vi "PH_IEEE1394Camera.get Bus Type.vi"(1 "Camera Attributes":T1[](array[typedef])) -> (0 "Bus Type":string)   [LabVIEW 2014, in "PH_IEEE1394Camera.lvlib"]
uses:
  PH_IEEE1394Camera.lvlib
  PH_IEEE1394Camera.Cam Attribute.ctl
  <vilib>/vision/driver/IMAQdx.llb/IMAQdx Attribute Type.ctl
  <vilib>/vision/driver/NI_Vision_Acquisition_Software.lvlib
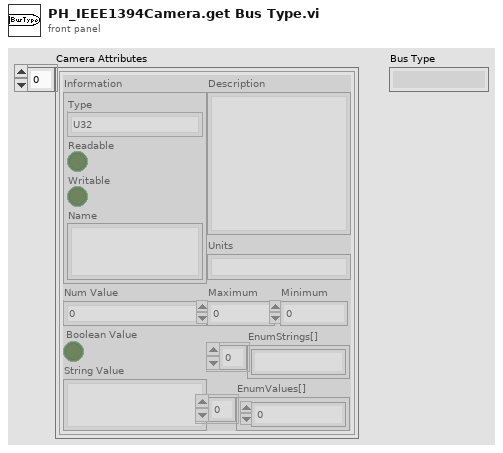
[diagram p1: front panel]
types:
  T1 = typedef "PH_IEEE1394Camera.lvlib/PH_IEEE1394Camera.Cam Attribute.ctl" = cluster{"Information":cluster{"Type":T2, "Readable":bool, "Writable":bool, "Name":string}, "Num Value":dbl, "String Value":string, "Maximum":dbl, "Minimum":dbl, "Units":string, "Description":string, "EnumStrings[]":string[], "EnumValues[]":u32[], "Boolean Value":bool}
  T2 = typedef "NI_Vision_Acquisition_Software.lvlib/IMAQdx Attribute Type.ctl" = enum32{"U32", "I64", "DBL", "String", "Enum", "Bool", "Command"}
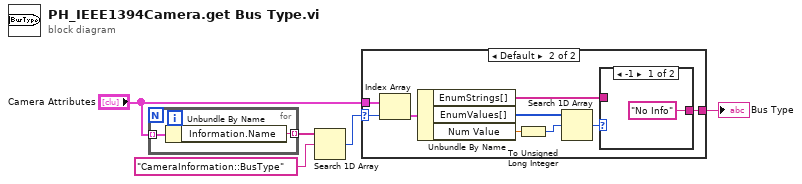
[diagram p0: block diagram]
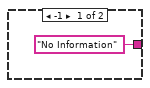
[diagram p2: hidden frame]
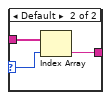
[diagram p3: hidden frame]
diagram:
  n1 = for {
    tunnel: "Camera Attributes" -> [w7] mode=indexing
    tunnel: [w6] -> w5 mode=indexing
    n2 = Unbundle By Name(w7) -> ("Information.Name"=w6:string)
  }
  n3 = Search 1D Array(1D array=w5, element="CameraInformation::BusType") -> (index of element=w1:i32)  [unwired: 1 in]
  n4 = case shown="Default" w1 {
    selector: w1 -> [_ w9]
    tunnel: "Camera Attributes" -> [_ w17]
    tunnel: ["No Information" w11] -> w2
    frame -1 {
    }
    frame Default {
      n5 = Index Array(array=w17, index=w9) -> (element=w16:T1)
      n6 = Unbundle By Name(w16) -> ("EnumStrings[]"=w15:string[], "EnumValues[]"=w14:u32[], "Num Value"=w13:dbl)
      n7 = To Unsigned Long Integer(number=w13) -> (unsigned 32bit integer=w12:u32)
      n8 = Search 1D Array(1D array=w14, element=w12) -> (index of element=w10:i32)  [unwired: 1 in]
      n9 = case shown="-1" w10 {
        selector: w10 -> [_ w19]
        tunnel: w15 -> [_ w21]
        tunnel: ["No Info" w20] -> w11
        frame -1 {
        }
        frame Default {
          n10 = Index Array(array=w21, index=w19) -> (element=w20:string)
        }
      }
    }
  }
  "Bus Type" <- w2
